vi "Actor Core.vi"(8 "error in":errorcluster, 11 "TRExperimentsRaw in":refnum<class "Sample Chemical Formula.lvclass">) -> (0 "error out":errorcluster, 3 "Actor out":refnum<class "Actor.lvclass">)   [LabVIEW 2020, in "Forms.lvlib" / "Sample Chemical Formula.lvclass"]
doc: "The user interface for this panel.\n\n----\nPlease see the following web address for additional documentation and tutorial information:\nhttp://www.mooregoodideas.com/mgi-panel-manager/\n\nAuthor: Derek Trepanier\n\nCopyright (c) 2018, Moore Good Ideas, Inc.\n\nAll rights reserved.\n\nRedistribution and use in source and binary forms, with or without modification, are permitted provided that the following conditions are met:\n\n * Redistributions of source code must retain the above copyright notice, this list of conditions and the following disclaimer.\n * Redistributions in binary form must reproduce the above copyright notice, this list of conditions and the following disclaimer in the documentation and/or other materials provided with the distribution.\n * Neither the name of Moore Good Ideas, Inc. nor the names of its contributors may be used to endorse or promote products derived from this software without specific prior written permission.\n\nTHIS SOFTWARE IS PROVIDED BY THE COPYRIGHT HOLDERS AND CONTRIBUTORS \"AS IS\" AND ANY EXPRESS OR IMPLIED WARRANTIES, INCLUDING, BUT NOT LIMITED TO, THE IMPLIED WARRANTIES OF MERCHANTABILITY AND FITNESS FOR A PARTICULAR PURPOSE ARE DISCLAIMED. IN NO EVENT SHALL THE COPYRIGHT OWNER OR CONTRIBUTORS BE LIABLE FOR ANY DIRECT, INDIRECT, INCIDENTAL, SPECIAL, EXEMPLARY, OR CONSEQUENTIAL DAMAGES (INCLUDING, BUT NOT LIMITED TO, PROCUREMENT OF SUBSTITUTE GOODS OR SERVICES; LOSS OF USE, DATA, OR PROFITS; OR BUSINESS INTERRUPTION) HOWEVER CAUSED AND ON ANY THEORY OF LIABILITY, WHETHER IN CONTRACT, STRICT LIABILITY, OR TORT (INCLUDING NEGLIGENCE OR OTHERWISE) ARISING IN ANY WAY OUT OF THE USE OF THIS SOFTWARE, EVEN IF ADVISED OF THE POSSIBILITY OF SUCH DAMAGE."
uses:
  Sample Chemical Formula.lvclass
  C:/Users/User/Desktop/Raman Program/Database OOP/source/Forms AF/Forms Controller/Form Controller/Panel Form Controller.lvclass
  <vilib>/ActorFramework/Actor/Actor.lvclass
  source/Forms AF/Forms Controller/Form Controller/Panel Form Controller.lvclass/Panel Form Controller.ctl
  source/Database OOP/Column Libraries/Basic Field Constructors/Text Field.vi
  source/Forms AF/Forms Controller/Form Window/Form Window.lvclass
  source/Database OOP/Table Libraries/Basic Form/Basic Form.lvclass
  source/Forms AF/Forms Controller/Form Controller/Panel Form Controller.lvclass
  source/Database OOP/Column Libraries/Composed Field Constructors.lvlib
panel:
  in  "Chemical Formula":string
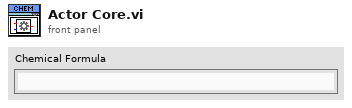
[diagram p1: front panel]
types:
  T1 = typedef "Panel Form Controller.lvlib/Builder Cluster.ctl" = cluster{"VI Ctrl Array":refnum<vi>[], "Form":refnum<class "Basic Form.lvclass">, "Open Form Button":refnum<class "Open Form Button.lvclass">}
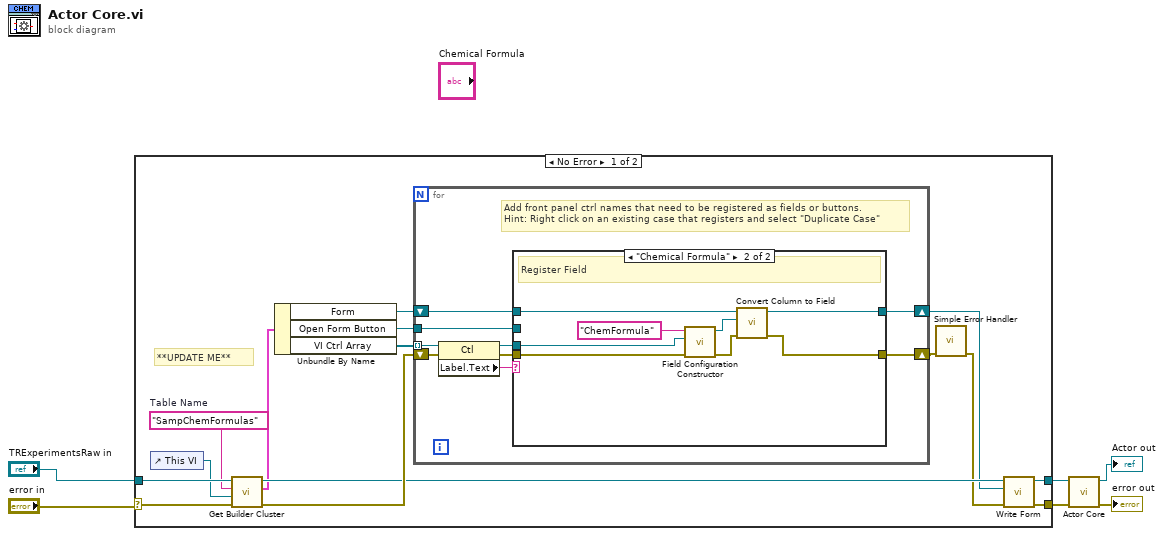
[diagram p0: block diagram]
diagram:
  n1 = case shown="No Error" "error in" {
    selector: "error in" -> [w18 w42]
    tunnel: "TRExperimentsRaw in" -> [w20 w41]
    tunnel: [w13 w42] -> w3
    tunnel: [w14 w41] -> w4
    frame No Error {
      w11 = "SampChemFormulas"  # Table Name
      # "**UPDATE ME**"
      n2 = control-ref of="This VI"() -> (w12:refnum<vi>)
      n3 = call "Get Builder Cluster.vi"("error in (no error)"=w18, "VI Refnum"=w12, "Table Name"=w11, "Panel Form Controller in"=w20) -> ("error out"=w19:errorcluster, "Builder Cluster"=w10:T1, "Panel Form Controller out"=w17:refnum<class "Sample Chemical Formula.lvclass">)  [unwired: 5 in]
      n4 = Unbundle By Name(w10) -> ("Form"=w7:refnum<class "Basic Form.lvclass">, "Open Form Button"=w8:refnum<class "Open Form Button.lvclass">, "VI Ctrl Array"=w9:refnum<vi>[])
      n5 = for {
        tunnel: w9 -> [w30] mode=indexing
        shift-right: [w23] -> w15
        shift-left: w7 -> [w24]
        shift-right: [w28] -> w21
        shift-left: w19 -> [w27]
        tunnel: w8 -> [w22]
        # "Add front panel ctrl names that need to be registered as fields or buttons.\nHint: Right click on an existing case that registers and select \"Duplicate Case\""
        n6 = property class="Ctl"(reference=w30, error in=w27) -> (reference out=w29:refnum<vi>, error out=w26:errorcluster, "Label.Text"=w25:string)
        n7 = case shown="\"Chemical Formula\"" w25 {
          tunnel: w29 -> [_ w35]
          tunnel: w24 -> [w32 w40]
          tunnel: [w32 w38] -> w23
          tunnel: [w31 w39] -> w28
          tunnel: w26 -> [w31 w34]
          tunnel: w22 -> [_ _]
          frame "", Default {
            # "Not Registered"
          }
          frame "Chemical Formula" {
            # "Register Field"
            n8 = call-poly "Field Configuration Constructor.vi"("error in"=w34, "Ctl Refnum"=w35, "Column Name"="ChemFormula" ("Column")) -> ("error out"=w37:errorcluster, "Field Configuration"=w33:refnum<class "Field Configuration.lvclass">)  [unwired: 7 in]
            n9 = call "Convert Column to Field.vi"("error in (no error)"=w37, "Field Configuration"=w33, "Basic Form in"=w40) -> ("error out"=w39:errorcluster, "Basic Form out"=w38:refnum<class "Basic Form.lvclass">)  [unwired: 7 in]
          }
        }
      }
      n10 = call <vilib>:"Simple Error Handler.vi"("error in (no error)"=w21) -> ("error out"=w16:errorcluster)  [unwired: 4 in, 4 out]
      n11 = call "Write Form.vi"("error in (no error)"=w16, "Form.lvlib:Basic Form.lvclass"=w15, "Panel Form Controller in"=w17) -> ("error out"=w13:errorcluster, "Panel Form Controller out"=w14:refnum<class "Sample Chemical Formula.lvclass">)  [unwired: 7 in]
    }
    frame Error {
    }
  }
  n12 = call-parent "Actor Core.vi"("error in"=w3, "Form Window in"=w4) -> ("error out"=→"error out":errorcluster, "Actor out"=→"Actor out":refnum<class "Actor.lvclass">)  [unwired: 8 in]
